vi "NanoXYZ_Monitor.vi"() -> ()   [LabVIEW 2012]
uses:
  Madlib.dll
  <vilib>/measure/NI_MABase.lvlib
panel:
  out "Z Position um":dbl(graph)
  in  "Z Offset um":dbl=50.0 min=0.0 max=200.0 step=1.0 format="%.3f"
  in  "Y Offset um":dbl=50.0 min=0.0 max=200.0 step=1.0 format="%.3f"
  out "Y Position um":dbl(graph)
  in  "signal type":T1(ring)
  in  "Amplitude (um)":dbl=10.0 min=0.0 max=100.0 step=0.1 format="%.3f"
  in  "X Offset um":dbl=50.0 min=0.0 max=200.0 step=1.0 format="%.3f"
  out "X Position um":dbl(graph)
  in  "?":bool
  # "This example VI demonstrates different types of motion on all axes ( Sine Wave, Triangle Wave, Square Wave\n, and Sawtooth Wave).  It outputs 100 data points per second on each axis.  Choosing a high frequency will lower \nthe amount of points per wave. For example a frequency of 5Hz will generate 5 sine waves in a second each \nconsisting of 20 data points."
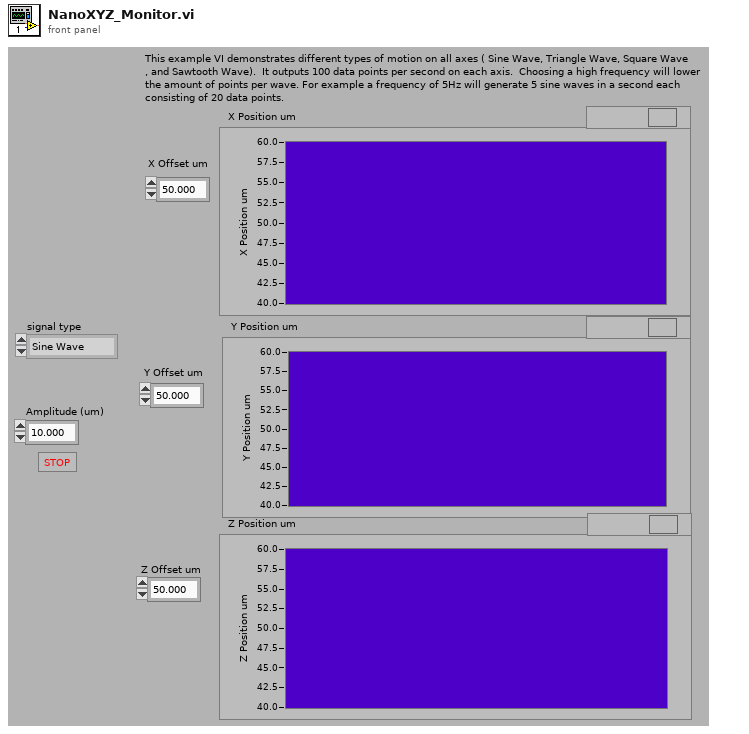
[diagram p1: front panel]
types:
  T1 = enum16{"Sine Wave", "Triangle Wave", "Square Wave", "Sawtooth Wave"}
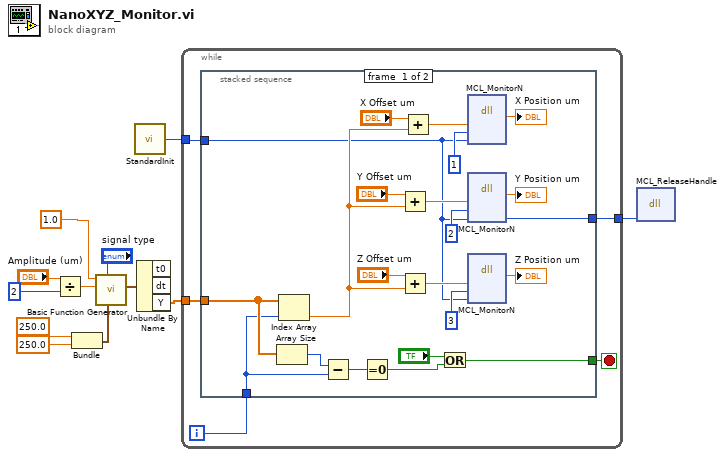
[diagram p0: block diagram]
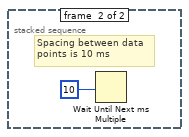
[diagram p2: hidden frame]
diagram:
  n1 = Divide(x="Amplitude (um)", y=2) -> (x/y=w8:dbl)
  n2 = Bundle(250.0, 250.0) -> (w10:cluster{dbl, dbl})  [unwired: 1 in]
  n3 = call <vilib>:"Basic Function Generator.vi"("sampling info"=w10, "signal type"="signal type", "amplitude"=w8, "frequency"=1.0) -> ("signal out"=w6:waveform(dbl))  [unwired: 5 in, 2 out]
  n4 = call "StandardInit.vi"() -> ("Outgoing Handle"=w2:i32)  [unwired: 1 in]
  n5 = Unbundle By Name ("Get Waveform Components")(w6) -> ("Y"=w4:dbl[])  [unwired: 2 out]
  n6 = while {
    tunnel: w4 -> [w17]
    tunnel: [w13] -> w3
    tunnel: w2 -> [w16]
    i -> [w15]
    stop <- w14 stop-if-true
    n7 = stacked-sequence {
      tunnel: w17 -> [w36 _]
      tunnel: w16 -> [w24 _]
      tunnel: w15 -> [w20 _]
      tunnel: [w19 _] -> w14
      tunnel: [w18 _] -> w13
      frame #0 {
        n8 = Array Size(array=w36) -> (size(s)=w39:i32)
        n9 = Index Array "Index Array"(array=w36, index=w20) -> (element=w28:dbl)
        n10 = Subtract(x=w39, y=w20) -> (x-y=w38:i32)
        n11 = Equal To 0?(x=w38) -> (x = 0?=w37:bool)
        n12 = Add(x="Y Offset um", y=w28) -> (x+y=w33:dbl)
        n13 = Add(x="Z Offset um", y=w28) -> (x+y=w32:dbl)
        n14 = Add(x="X Offset um", y=w28) -> (x+y=w34:dbl)
        n15 = Or(x="?", y=w37) -> (x .or. y?=w19:bool)
        n16 = dll-call lib="C:/Users/Labview/Desktop/SRR/Madlib_x64/Labview Examples/MADLib.dll" fn="MCL_MonitorN"("position"=w34, "axis"=u16 1, "handle"=w24) -> (→"X Position um":dbl)  [unwired: 6 in, 2 out]
        n17 = dll-call lib="C:/Users/Labview/Desktop/SRR/Madlib_x64/Labview Examples/MADLib.dll" fn="MCL_MonitorN"("position"=w33, "axis"=u16 2, "handle"=w24) -> (→"Y Position um":dbl, "handle"=w18:i32)  [unwired: 5 in, 2 out]
        n18 = dll-call lib="C:/Users/Labview/Desktop/SRR/Madlib_x64/Labview Examples/MADLib.dll" fn="MCL_MonitorN"("position"=w32, "axis"=3, "handle"=w24) -> (→"Z Position um":dbl)  [unwired: 6 in, 2 out]
      }
      frame #1 {
        # "Spacing between data\npoints is 10 ms"
        n19 = Wait Until Next ms Multiple(millisecond multiple=10) -> ()  [unwired: 1 out]
      }
    }
  }
  n20 = dll-call lib="C:/Users/Labview/Desktop/SRR/Madlib_x64/Labview Examples/MADLib.dll" fn="MCL_ReleaseHandle"("handle"=w3) -> ()  [unwired: 5 in, 2 out]
